vi "CRYProtect All.vi"(8 "sNames":string[](array[string]), 9 "sOption":string, 10 "Index":i32[](array[numeric]), 11 "Type":enum16{"Curves", "Values", "Results", "WFM"}(ring)) -> (0 "Inserted Index":i32[](array[numeric]), 1 "Protect?":bool=TRUE, 2 "Protected Rows":i32[](array[numeric]), 3 "Protected NewNames":string[](array[string]), 4 "Protected OrgNames":string[](array[string]))   [LabVIEW 2013]
uses:
  Global/CRYCurve Library Global.vi
panel:
  # "Prodect All Data(Curves, Values, Results, Waveforms)"
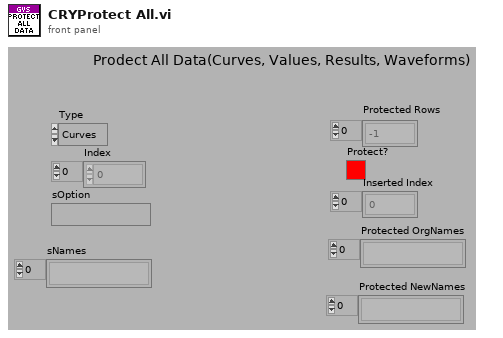
[diagram p1: front panel]
types:
  T1 = enum16{"OK", "Yes", "YesNo", "YesNoCancel", "ReplaceAppend"}
  T2 = cluster{"Curve OrgNames":string[], "Value OrgNames":string[], "Result OrgNames":string[], "WFM OrgNames":string[], "Curve NewNames":string[], "Value NewNames":string[], "Result NewNames":string[], "WFM NewNames":string[]}
  T3 = cluster{"Curve Index":i32[], "Value Index":i32[], "Result Index":i32[], "WFM Index":i32[], "Curve Names":string[], "Value Names":string[], "Result Names":string[], "WFM Names":string[]}
  T4 = typedef "CRYWaveform Cluster Array.ctl" = T5[]
  T5 = typedef "CRYWaveform Cluster.ctl" = cluster{"Waveform":cluster{"X0":dbl, "dX":dbl, "Y":sgl[]}, "X data":u16, "Y data":u16, "Y axis":u16, "X unit":string, "Y unit":string, "Y dB ref":dbl, "display Y":bool, "display X":bool, "Overload?":bool, "Test Info":string, "Step No.":i32, "Name":string, "protected":bool, "Sqc history":string[], "Signal Channel ID":i32, "Plot Settings":cluster{"Color":u32, "Interpolation":u8, "Point Style":u8, "Line Style":u8, "Point Color":u32, "Line Width":u8, "Bar Plot Style":u8, "Fill To":i16}, "AutoProtect":bool}
  T6 = typedef "CRYResult Cluster Array.ctl" = T7[]
  T7 = typedef "CRYResult Cluster.ctl" = cluster{"Name":string, "Margin":dbl, "unit":string, "Verdict":bool, "Limit":string, "Max/Min":string, "protected":bool, "Step No.":i32, "Test Info":string, "AutoProtect":bool}
  T8 = typedef "CRYData Cluster Array.ctl" = T9[]
  T9 = typedef "CRYData Cluster.ctl" = cluster{"Name":string, "Curve":cluster{"x":dbl, "y":dbl, "z":dbl}[], "X data":u16, "Y data":u16, "Z data":u16, "X axis":u16, "Y axis":u16, "Z axis":u16, "X unit":string, "Y unit":string, "Z unit":string, "X dB ref":dbl, "Y dB ref":dbl, "Z dB ref":dbl, "single val":bool, "protected":bool, "display X":bool, "display Y":bool, "display Z":bool, "Test Info":string, "Step No.":i32, "Plot Settings":cluster{"Color":u32, "Interpolation":u8, "Point Style":u8, "Line Style":u8, "Point Color":u32, "Line Width":u8, "Bar Plot Style":u8, "Fill To":i16}, "AutoProtect":bool}
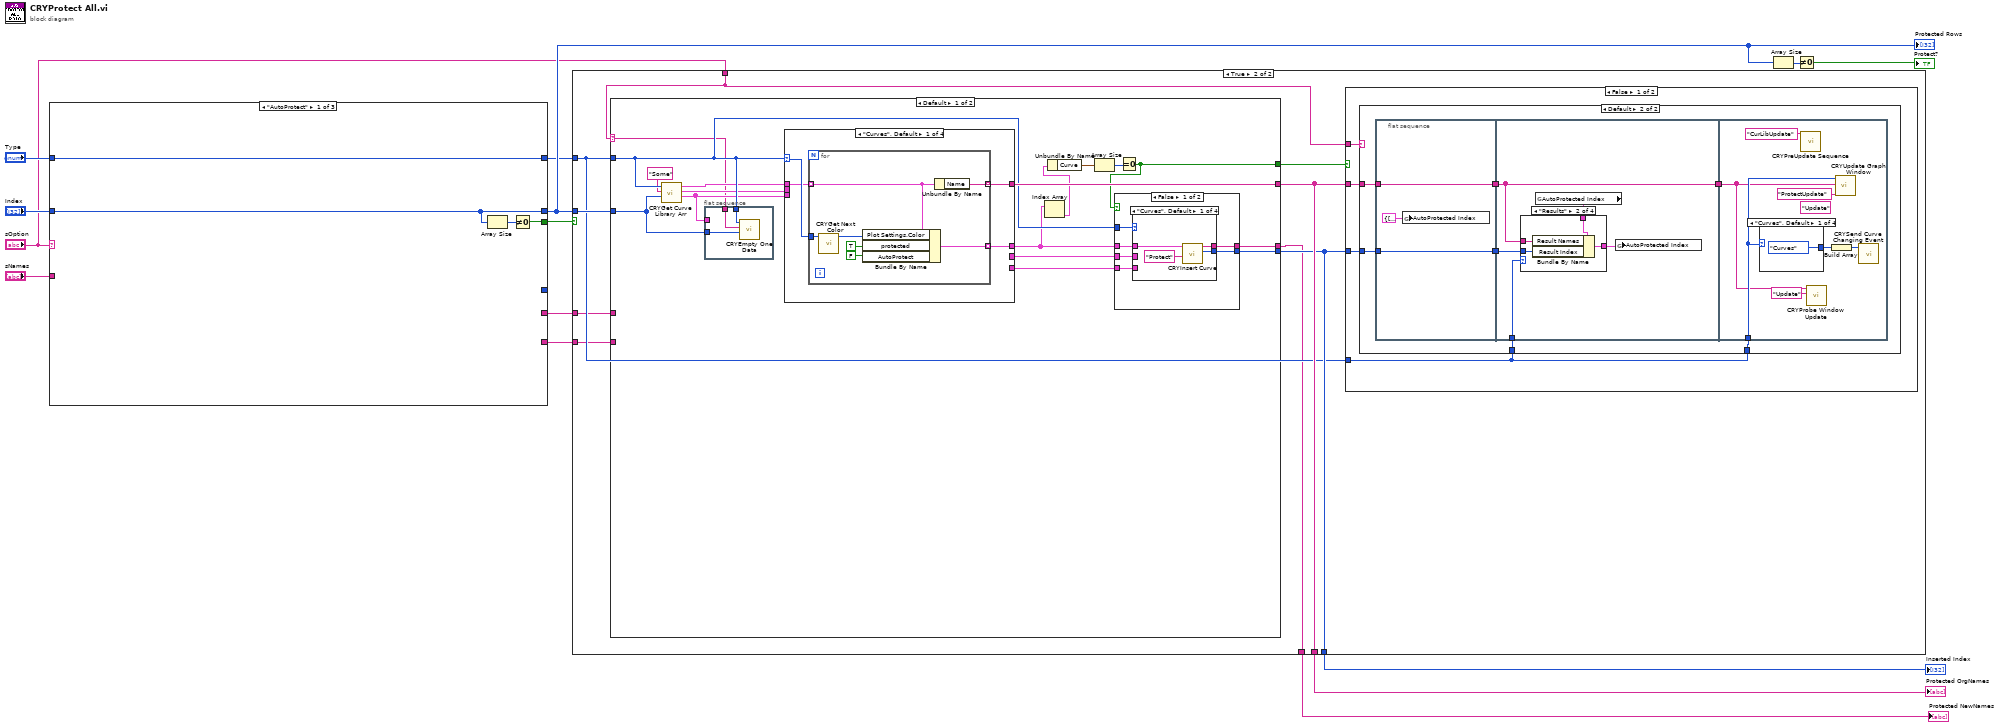
[diagram p0: block diagram]
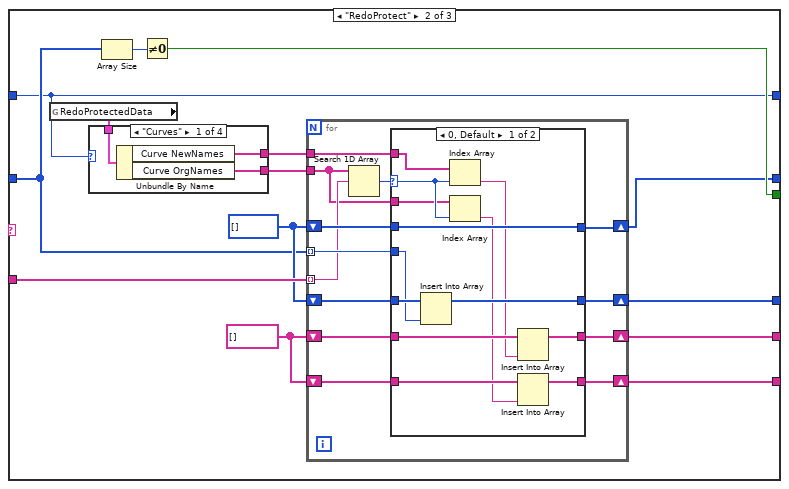
[diagram p2: hidden frame]
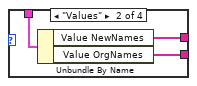
[diagram p3: hidden frame]
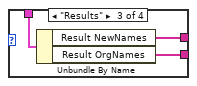
[diagram p4: hidden frame]
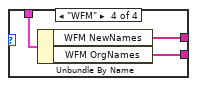
[diagram p5: hidden frame]
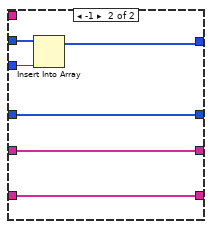
[diagram p6: hidden frame]
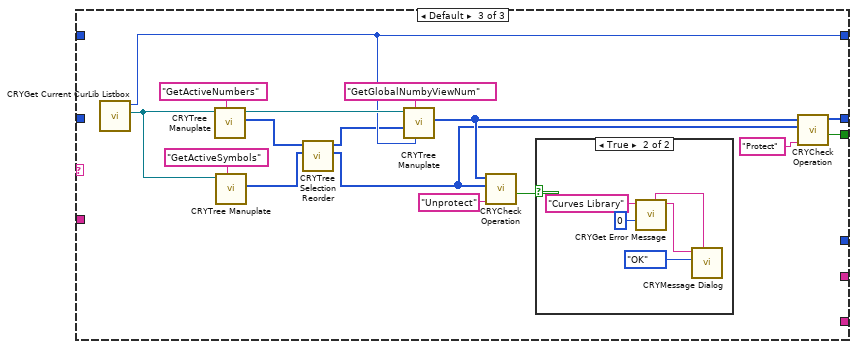
[diagram p7: hidden frame]
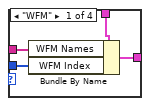
[diagram p11: hidden frame]
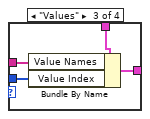
[diagram p12: hidden frame]
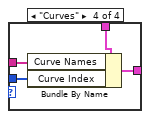
[diagram p13: hidden frame]
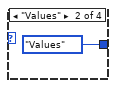
[diagram p14: hidden frame]
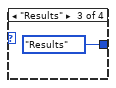
[diagram p15: hidden frame]
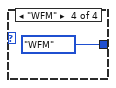
[diagram p16: hidden frame]
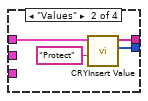
[diagram p18: hidden frame]
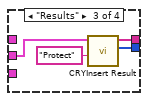
[diagram p19: hidden frame]
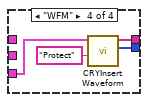
[diagram p20: hidden frame]
diagram:
  n1 = case shown="\"AutoProtect\"" "sOption" {
    tunnel: [w15 w31 w88] -> w14
    tunnel: [w17 w25 w89] -> w13
    tunnel: [w18 w19 w81] -> w10
    tunnel: "Type" -> [w18 w19 _]
    tunnel: "Index" -> [w17 w26 _]
    tunnel: "sNames" -> [_ w28 _]
    tunnel: [_ w24 _] -> _
    tunnel: [_ w23 _] -> w3
    tunnel: [_ w20 _] -> w2
    frame "AutoProtect" {
      n2 = Array Size(array=w17) -> (size(s)=w16:i32)
      n3 = Not Equal To 0?(x=w16) -> (x != 0?=w15:bool)
    }
    frame "RedoProtect" {
      w21 = string[] [] ("sNames")
      w27 = i32[] [] ("Index")
      n4 = global read "CRYCurve Library Global.vi" "RedoProtectedData"() -> (w30:T2)
      n5 = case shown="\"Curves\"" w19 {
        tunnel: w30 -> [w35 w38 w41 w44]
        tunnel: [w34 w37 w40 w43] -> w29
        tunnel: [w33 w36 w39 w42] -> w22
        frame "Curves" {
          n6 = Unbundle By Name(w35) -> ("Curve NewNames"=w33:string[], "Curve OrgNames"=w34:string[])
        }
        frame "Values" {
          n7 = Unbundle By Name(w38) -> ("Value NewNames"=w36:string[], "Value OrgNames"=w37:string[])
        }
        frame "Results" {
          n8 = Unbundle By Name(w41) -> ("Result NewNames"=w39:string[], "Result OrgNames"=w40:string[])
        }
        frame "WFM" {
          n9 = Unbundle By Name(w44) -> ("WFM NewNames"=w42:string[], "WFM OrgNames"=w43:string[])
        }
      }
      n10 = Array Size(array=w26) -> (size(s)=w32:i32)
      n11 = Not Equal To 0?(x=w32) -> (x != 0?=w31:bool)
      n12 = for {
        tunnel: w29 -> [w46]
        tunnel: w28 -> [w49] mode=indexing
        tunnel: w26 -> [w56] mode=indexing
        shift-right: [w54] -> w25
        shift-left: w27 -> [w55]
        shift-right: [w52] -> w24
        shift-left: w27 -> [w53]
        shift-right: [w50] -> w23
        shift-left: w21 -> [w51]
        tunnel: w22 -> [w48]
        shift-right: [w45] -> w20
        shift-left: w21 -> [w47]
        n13 = Search 1D Array(1D array=w46, element=w49) -> (index of element=w57:i32)  [unwired: 1 in]
        n14 = case shown="0, Default" w57 {
          selector: w57 -> [w61 _]
          tunnel: w56 -> [w67 w75]
          tunnel: w55 -> [w70 w76]
          tunnel: [w70 w74] -> w54
          tunnel: w53 -> [w69 w73]
          tunnel: [w68 w73] -> w52
          tunnel: w51 -> [w66 w72]
          tunnel: [w65 w72] -> w50
          tunnel: w48 -> [w64 _]
          tunnel: w47 -> [w62 w71]
          tunnel: w46 -> [w60 _]
          tunnel: [w58 w71] -> w45
          frame 0, Default {
            n15 = Insert Into Array(array=w69, new element=w67) -> (w68:i32[])  [unwired: 1 in]
            n16 = Index Array(array=w64, index=w61) -> (element=w63:string)
            n17 = Index Array(array=w60, index=w61) -> (element=w59:string)
            n18 = Insert Into Array(array=w66, new element=w63) -> (w65:string[])  [unwired: 1 in]
            n19 = Insert Into Array(array=w62, new element=w59) -> (w58:string[])  [unwired: 1 in]
          }
          frame -1 {
            n20 = Insert Into Array(array=w76, new element=w75) -> (w74:i32[])  [unwired: 1 in]
          }
        }
      }
    }
    frame Default {
      n21 = call "CRYGet Current CurLib Listbox.vi"() -> ("CurLib Tree"=w85:refnum<vi>, "Type"=w81:enum16{"Curves", "Values", "Results", "WFM"})  [unwired: 9 in, 1 out]
      n22 = call "CRYTree Manuplate.vi"("sAction"="GetActiveNumbers", "Tree in"=w85) -> ("nData Out"=w80:i32[], "Tree Out"=w83:refnum<vi>)  [unwired: 6 in, 2 out]
      n23 = call "CRYTree Manuplate.vi"("sAction"="GetActiveSymbols", "Tree in"=w85) -> ("nData Out"=w78:i32[])  [unwired: 6 in, 3 out]
      n24 = call "CRYTree Selection Reorder.vi"("Symbol In"=w78, "Number In"=w80) -> ("Symbol Out"=w77:i32[], "Number Out"=w79:i32[])  [unwired: 8 in]
      n25 = call "CRYTree Manuplate.vi"("Type"=w81, "sAction"="GetGlobalNumbyViewNum", "nData"=w79, "Tree in"=w83) -> ("nData Out"=w82:i32[])  [unwired: 4 in, 3 out]
      n26 = call "CRYCheck Operation.vi"("Operation"="Unprotect", "Item Symbols In"=w77, "Index Array In"=w82) -> ("Operation ?"=w92:bool)  [unwired: 6 in, 2 out]
      n27 = case shown="True" w92 {
        frame False {
        }
        frame True {
          n28 = call "CRYGet Error Message.vi"("Error No"=0, "Kind"="Curves Library") -> ("Message"=w94:string, "Window Title"=w93:string)  [unwired: 4 in, 4 out]
          n29 = call "CRYMessage Dialog.vi"("Window Title"=w93, "YesNoCancel"=T1."OK", "Message Content"=w94) -> ()  [unwired: 7 in, 2 out]
        }
      }
      n30 = call "CRYCheck Operation.vi"("Operation"="Protect", "Item Symbols In"=w77, "Index Array In"=w82) -> ("Operation ?"=w88:bool, "Array Out"=w89:i32[])  [unwired: 6 in, 1 out]
    }
  }
  "Protected Rows" <- w13
  n31 = case shown="True" w14 {
    tunnel: w13 -> [_ w106]
    tunnel: w10 -> [_ w103]
    tunnel: "sOption" -> [_ w102]
    tunnel: [_ w104] -> w7
    tunnel: [_ w105] -> w6
    tunnel: w3 -> [_ w101]
    tunnel: w2 -> [_ w100]
    tunnel: [_ w99] -> w1
    frame False {
    }
    frame True {
      n32 = case shown="Default" w102 {
        selector: w102 -> [w159 w245]
        tunnel: w106 -> [w169 w253]
        tunnel: [w168 w234] -> w105
        tunnel: [w167 w235] -> w104
        tunnel: w103 -> [w166 w238]
        tunnel: w101 -> [_ w236]
        tunnel: w100 -> [_ w240]
        tunnel: [w158 w233] -> w99
        tunnel: [w153 _] -> w98
        frame Default {
          n33 = call "CRYGet Curve Library Arr.vi"("Index"=w169, "sOption"="Some", "Type In"=w166) -> ("Waveforms"=w160:T4, "Results"=w164:T6, "Curves/Values"=w165:T8)  [unwired: 6 in]
          n34 = flat-sequence {
            tunnel: w169 -> [w194]
            tunnel: w159 -> [w193]
            tunnel: w166 -> [w192]
            tunnel: w160 -> [_]
            frame #0 {
              n35 = call "CRYEmpty One Data.vi"("Index"=w194, "sOption"=w193, "Type"=w192) -> ()  [unwired: 9 out]
            }
          }
          n36 = case shown="\"Curves\", Default" w166 {
            selector: w166 -> [w197 _ _ w224]
            tunnel: [w198 w208 w216 w225] -> w168
            tunnel: w165 -> [w196 w207 _ _]
            tunnel: w164 -> [_ _ w215 _]
            tunnel: w160 -> [_ _ _ w223]
            tunnel: [w195 w206 _ _] -> w157
            tunnel: [_ _ w214 _] -> w162
            tunnel: [_ _ _ w222] -> w161
            frame "Curves", Default {
              n37 = for {
                tunnel: [w204] -> w198 mode=indexing
                tunnel: w197 -> [w202]
                tunnel: w196 -> [w200] mode=indexing
                tunnel: [w199] -> w195 mode=indexing
                n38 = call "CRYGet Next Color.vi"("Type"=w202) -> ("Color"=w201:u32)  [unwired: 10 out]
                n39 = Bundle By Name(cluster=w200, "Plot Settings.Color"=w201, "protected"=TRUE, "AutoProtect"=FALSE ("protected")) -> (w199:T9)
                n40 = Unbundle By Name(w200) -> ("Name"=w204:string)
              }
            }
            frame "Values" {
              n41 = for {
                tunnel: [w212] -> w208 mode=indexing
                tunnel: w207 -> [w210] mode=indexing
                tunnel: [w209] -> w206 mode=indexing
                n42 = Bundle By Name(cluster=w210, "protected"=TRUE, "AutoProtect"=FALSE) -> (w209:T9)
                n43 = Unbundle By Name(w210) -> ("Name"=w212:string)
              }
            }
            frame "Results" {
              n44 = for {
                tunnel: [w220] -> w216 mode=indexing
                tunnel: w215 -> [w218] mode=indexing
                tunnel: [w217] -> w214 mode=indexing
                n45 = Bundle By Name(cluster=w218, "protected"=TRUE, "AutoProtect"=FALSE) -> (w217:T7)
                n46 = Unbundle By Name(w218) -> ("Name"=w220:string)
              }
            }
            frame "WFM" {
              n47 = for {
                tunnel: [w231] -> w225 mode=indexing
                tunnel: w224 -> [w229]
                tunnel: w223 -> [w227] mode=indexing
                tunnel: [w226] -> w222 mode=indexing
                n48 = call "CRYGet Next Color.vi"("Type"=w229) -> ("Color"=w228:u32)  [unwired: 10 out]
                n49 = Bundle By Name(cluster=w227, "Plot Settings.Color"=w228, "protected"=TRUE, "AutoProtect"=FALSE) -> (w226:T5)
                n50 = Unbundle By Name(w227) -> ("Name"=w231:string)
              }
            }
          }
          n51 = Index Array(array=w157) -> (element=w156:T9)  [unwired: 1 in]
          n52 = Unbundle By Name(w156) -> ("Curve"=w155:cluster{"x":dbl, "y":dbl, "z":dbl}[])
          n53 = Array Size(array=w155) -> (size(s)=w154:i32)
          n54 = Equal To 0?(x=w154) -> (x = 0?=w153:bool)
          n55 = case shown="False" w153 {
            tunnel: [w175 _] -> w167
            tunnel: w166 -> [w174 _]
            tunnel: w162 -> [w173 _]
            tunnel: w161 -> [w172 _]
            tunnel: [w171 _] -> w158
            tunnel: w157 -> [w170 _]
            frame False {
              n56 = case shown="\"Curves\", Default" w174 {
                tunnel: w170 -> [w178 w182 _ _]
                tunnel: [w177 w181 w186 w190] -> w175
                tunnel: w173 -> [_ _ w185 _]
                tunnel: w172 -> [_ _ _ w189]
                tunnel: [w176 w180 w184 w188] -> w171
                frame "Curves", Default {
                  n57 = call "CRYInsert Curve.vi"("sOption"="Protect", "Curve"=w178) -> ("Inserted Index"=w177:i32[], "Inserted Name Out"=w176:string[])  [unwired: 2 in, 6 out]
                }
                frame "Values" {
                  n58 = call "CRYInsert Value.vi"("sOption"="Protect", "Value"=w182) -> ("Inserted Index"=w181:i32[], "Inserted Name Out"=w180:string[])  [unwired: 8 in]
                }
                frame "Results" {
                  n59 = call "CRYInsert Result.vi"("sOption"="Protect", "Result"=w185) -> ("Inserted Index"=w186:i32[], "Inserted Name Out"=w184:string[])  [unwired: 8 in]
                }
                frame "WFM" {
                  n60 = call "CRYInsert Waveform.vi"("sOption"="Protect", "Waveform"=w189) -> ("Inserted Index"=w190:i32[], "Inserted Name Out"=w188:string[])  [unwired: 8 in]
                }
              }
            }
            frame True {
            }
          }
        }
        frame "RedoProtect" {
          n61 = flat-sequence {
            tunnel: w245 -> [w327]
            tunnel: w238 -> [w324]
            tunnel: w240 -> [w326]
            tunnel: w239 -> [_]
            frame #0 {
              n62 = for {
                tunnel: w324 -> [w330]
                tunnel: w326 -> [w329] mode=indexing
                tunnel: [w328] -> w325 mode=indexing
                n63 = call "CRYGet Curve Library One Data .vi"("Data Name"=w329, "Type"=w330) -> ("index"=w328:i32)  [unwired: 3 in, 6 out]
              }
              n64 = call "CRYEmpty One Data.vi"("Index"=w325, "sOption"=w327, "Type"=w324) -> ()  [unwired: 9 out]
            }
          }
          n65 = flat-sequence {
            tunnel: w253 -> [w266]
            tunnel: [w265] -> w234
            tunnel: [w264] -> w235
            tunnel: w245 -> [w256]
            tunnel: w237 -> [w255]
            tunnel: [w254] -> w233
            frame #0 {
              n66 = call "CRYGet Curve Library Arr.vi"("Index"=w266, "sOption"="Some", "Type In"=w255) -> ("Waveforms"=w257:T4, "Results"=w262:T6, "Curves/Values"=w263:T8)  [unwired: 6 in]
              n67 = flat-sequence {
                tunnel: w266 -> [w269]
                tunnel: w256 -> [w268]
                tunnel: w255 -> [w267]
                tunnel: w257 -> [_]
                frame #0 {
                  n68 = call "CRYEmpty One Data.vi"("Index"=w269, "sOption"=w268, "Type"=w267) -> ()  [unwired: 9 out]
                }
              }
              n69 = case shown="\"WFM\"" w255 {
                selector: w255 -> [w272 _ _ w299]
                tunnel: [w273 w283 w291 w300] -> w265
                tunnel: w263 -> [w271 w282 _ _]
                tunnel: w262 -> [_ _ w290 _]
                tunnel: w257 -> [_ _ _ w298]
                tunnel: [w270 w281 _ _] -> w260
                tunnel: [_ _ w289 _] -> w259
                tunnel: [_ _ _ w297] -> w258
                frame "Curves", Default {
                  n70 = for {
                    tunnel: [w279] -> w273 mode=indexing
                    tunnel: w272 -> [w277]
                    tunnel: w271 -> [w275] mode=indexing
                    tunnel: [w274] -> w270 mode=indexing
                    n71 = call "CRYGet Next Color.vi"("Type"=w277) -> ("Color"=w276:u32)  [unwired: 10 out]
                    n72 = Bundle By Name(cluster=w275, "Plot Settings.Color"=w276, "protected"=TRUE, "AutoProtect"=FALSE ("protected")) -> (w274:T9)
                    n73 = Unbundle By Name(w275) -> ("Name"=w279:string)
                  }
                }
                frame "Values" {
                  n74 = for {
                    tunnel: [w287] -> w283 mode=indexing
                    tunnel: w282 -> [w285] mode=indexing
                    tunnel: [w284] -> w281 mode=indexing
                    n75 = Bundle By Name(cluster=w285, "protected"=TRUE, "AutoProtect"=FALSE) -> (w284:T9)
                    n76 = Unbundle By Name(w285) -> ("Name"=w287:string)
                  }
                }
                frame "Results" {
                  n77 = for {
                    tunnel: [w295] -> w291 mode=indexing
                    tunnel: w290 -> [w293] mode=indexing
                    tunnel: [w292] -> w289 mode=indexing
                    n78 = Bundle By Name(cluster=w293, "protected"=TRUE, "AutoProtect"=FALSE) -> (w292:T7)
                    n79 = Unbundle By Name(w293) -> ("Name"=w295:string)
                  }
                }
                frame "WFM" {
                  n80 = for {
                    tunnel: [w306] -> w300 mode=indexing
                    tunnel: w299 -> [w304]
                    tunnel: w298 -> [w302] mode=indexing
                    tunnel: [w301] -> w297 mode=indexing
                    n81 = call "CRYGet Next Color.vi"("Type"=w304) -> ("Color"=w303:u32)  [unwired: 10 out]
                    n82 = Bundle By Name(cluster=w302, "Plot Settings.Color"=w303, "protected"=TRUE, "AutoProtect"=FALSE) -> (w301:T5)
                    n83 = Unbundle By Name(w302) -> ("Name"=w306:string)
                  }
                }
              }
              n84 = case shown="\"WFM\"" w255 {
                tunnel: w260 -> [w310 w314 _ _]
                tunnel: [w309 w313 w318 w322] -> w264
                tunnel: w259 -> [_ _ w317 _]
                tunnel: w258 -> [_ _ _ w321]
                tunnel: [w308 w312 w316 w320] -> w254
                frame "Curves", Default {
                  n85 = call "CRYInsert Curve.vi"("sOption"="Protect", "Curve"=w310) -> ("Inserted Index"=w309:i32[], "Inserted Name Out"=w308:string[])  [unwired: 2 in, 6 out]
                }
                frame "Values" {
                  n86 = call "CRYInsert Value.vi"("sOption"="Protect", "Value"=w314) -> ("Inserted Index"=w313:i32[], "Inserted Name Out"=w312:string[])  [unwired: 8 in]
                }
                frame "Results" {
                  n87 = call "CRYInsert Result.vi"("sOption"="Protect", "Result"=w317) -> ("Inserted Index"=w318:i32[], "Inserted Name Out"=w316:string[])  [unwired: 8 in]
                }
                frame "WFM" {
                  n88 = call "CRYInsert Waveform.vi"("sOption"="Protect", "Waveform"=w321) -> ("Inserted Index"=w322:i32[], "Inserted Name Out"=w320:string[])  [unwired: 8 in]
                }
              }
            }
          }
          n89 = call "CRYGlobal Manipulate.vi"("Type"=w238, "sOption"="byNames", "sAction"="GetGlobal", "sData"=w236) -> ("Curves Out"=w250:T9[], "Values Out"=w249:T9[], "WFM Out"=w247:T5[], "Results Out"=w248:T7[])  [unwired: 5 in, 3 out]
          n90 = call "CRYGlobal Manipulate.vi"("Type"=w238, "sOption"="byNames", "sAction"="GetGlobal", "sData"=w240) -> ("Curves Out"=w243:T9[], "Values Out"=w242:T9[], "WFM Out"=w239:T5[], "Results Out"=w241:T7[])  [unwired: 5 in, 3 out]
          n91 = case shown="\"Curves\", Default" w238 {
            selector: w238 -> [w331 w360 w386 w403]
            tunnel: w250 -> [w337 _ _ _]
            tunnel: w249 -> [_ w358 _ _]
            tunnel: w248 -> [_ _ w385 _]
            tunnel: w247 -> [_ _ _ w402]
            tunnel: w243 -> [w336 _ _ _]
            tunnel: w242 -> [_ w357 _ _]
            tunnel: w241 -> [_ _ w384 _]
            tunnel: w239 -> [_ _ _ w401]
            tunnel: w236 -> [w333 w361 w387 w404]
            tunnel: [w331 w360 w386 w403] -> w237
            frame "Curves", Default {
              n92 = for {
                tunnel: w337 -> [w340] mode=indexing
                tunnel: [w339] -> w332 mode=indexing
                tunnel: w336 -> [w338] mode=indexing
                n93 = Unbundle By Name(w338) -> ("Curve"=w356:cluster{"x":dbl, "y":dbl, "z":dbl}[], "X data"=w355:u16, "Y data"=w354:u16, "Z data"=w353:u16, "X axis"=w352:u16, "Y axis"=w351:u16, "Z axis"=w350:u16, "X unit"=w349:string, "Y unit"=w348:string, "Z unit"=w347:string, "X dB ref"=w346:dbl, "Y dB ref"=w345:dbl, "Z dB ref"=w344:dbl, "display X"=w343:bool, "display Y"=w342:bool, "display Z"=w341:bool)
                n94 = Bundle By Name(cluster=w340, "Curve"=w356, "X data"=w355, "Y data"=w354, "Z data"=w353, "X axis"=w352, "Y axis"=w351, "Z axis"=w350, "X unit"=w349, "Y unit"=w348, "Z unit"=w347, "X dB ref"=w346, "Y dB ref"=w345, "Z dB ref"=w344, "display X"=w343, "display Y"=w342, "display Z"=w341) -> (w339:T9)
              }
              n95 = call "CRYGlobal Manipulate.vi"("Type"=w331, "sOption"="byNames", "sAction"="Replace", "sData"=w333, "Curves"=w332) -> ()  [unwired: 4 in, 7 out]
            }
            frame "Values" {
              n96 = for {
                tunnel: w358 -> [w366] mode=indexing
                tunnel: [w365] -> w359 mode=indexing
                tunnel: w357 -> [w364] mode=indexing
                n97 = Unbundle By Name(w364) -> ("Curve"=w382:cluster{"x":dbl, "y":dbl, "z":dbl}[], "X data"=w381:u16, "Y data"=w380:u16, "Z data"=w379:u16, "X axis"=w378:u16, "Y axis"=w377:u16, "Z axis"=w376:u16, "X unit"=w375:string, "Y unit"=w374:string, "Z unit"=w373:string, "X dB ref"=w372:dbl, "Y dB ref"=w371:dbl, "Z dB ref"=w370:dbl, "display X"=w369:bool, "display Y"=w368:bool, "display Z"=w367:bool)
                n98 = Bundle By Name(cluster=w366, "Curve"=w382, "X data"=w381, "Y data"=w380, "Z data"=w379, "X axis"=w378, "Y axis"=w377, "Z axis"=w376, "X unit"=w375, "Y unit"=w374, "Z unit"=w373, "X dB ref"=w372, "Y dB ref"=w371, "Z dB ref"=w370, "display X"=w369, "display Y"=w368, "display Z"=w367) -> (w365:T9)
              }
              n99 = call "CRYGlobal Manipulate.vi"("Type"=w360, "sOption"="byNames", "sAction"="Replace", "sData"=w361, "Values"=w359) -> ()  [unwired: 4 in, 7 out]
            }
            frame "Results" {
              n100 = for {
                tunnel: w385 -> [w399] mode=indexing
                tunnel: [w398] -> w383 mode=indexing
                tunnel: w384 -> [w397] mode=indexing
                n101 = Unbundle By Name(w397) -> ("Margin"=w396:dbl, "unit"=w395:string, "Verdict"=w394:bool, "Limit"=w393:string, "Max/Min"=w392:string, "Step No."=w391:i32, "Test Info"=w390:string)
                n102 = Bundle By Name(cluster=w399, "Margin"=w396, "unit"=w395, "Verdict"=w394, "Limit"=w393, "Max/Min"=w392, "Step No."=w391, "Test Info"=w390) -> (w398:T7)
              }
              n103 = call "CRYGlobal Manipulate.vi"("Type"=w386, "sOption"="byNames", "sAction"="Replace", "sData"=w387, "Results"=w383) -> ()  [unwired: 4 in, 7 out]
            }
            frame "WFM" {
              n104 = for {
                tunnel: w402 -> [w423] mode=indexing
                tunnel: [w422] -> w400 mode=indexing
                tunnel: w401 -> [w421] mode=indexing
                n105 = Unbundle By Name(w421) -> ("Waveform"=w420:cluster{"X0":dbl, "dX":dbl, "Y":sgl[]}, "X data"=w419:u16, "Y data"=w418:u16, "Y axis"=w417:u16, "X unit"=w416:string, "Y unit"=w415:string, "Y dB ref"=w414:dbl, "display Y"=w413:bool, "display X"=w412:bool, "Overload?"=w411:bool, "Test Info"=w410:string, "Step No."=w409:i32, "Sqc history"=w408:string[], "Signal Channel ID"=w407:i32)
                n106 = Bundle By Name(cluster=w423, "Waveform"=w420, "X data"=w419, "Y data"=w418, "Y axis"=w417, "X unit"=w416, "Y unit"=w415, "Y dB ref"=w414, "display Y"=w413, "display X"=w412, "Overload?"=w411, "Test Info"=w410, "Step No."=w409, "Sqc history"=w408, "Signal Channel ID"=w407) -> (w422:T5)
              }
              n107 = call "CRYGlobal Manipulate.vi"("Type"=w403, "sOption"="byNames", "sAction"="Replace", "sData"=w404, "WFM"=w400) -> ()  [unwired: 4 in, 7 out]
            }
          }
        }
      }
      n108 = case shown="False" w98 {
        tunnel: w105 -> [w110 _]
        tunnel: w104 -> [w109 _]
        tunnel: w103 -> [w108 _]
        tunnel: w102 -> [w107 _]
        frame False {
          n109 = case shown="Default" w107 {
            tunnel: w110 -> [_ w117]
            tunnel: w109 -> [_ w115]
            tunnel: w108 -> [_ w112]
            tunnel: w108 -> [_ w111]
            frame "AutoProtect", "RedoProtect" {
              # "In Sequence Run or Redo , donot update curvelibgraph"
            }
            frame Default {
              n110 = flat-sequence {
                tunnel: w115 -> [w119]
                tunnel: w117 -> [w120]
                tunnel: [w120] -> w114
                tunnel: [w119] -> w113
                tunnel: [w121] -> w116
                tunnel: w114 -> [w121]
                tunnel: w113 -> [w123]
                tunnel: w111 -> [w122]
                tunnel: w116 -> [w142]
                tunnel: w112 -> [w143]
                frame #0 {
                  n111 = global write "CRYCurve Library Global.vi" "AutoProtected Index"(T3 {"Curve Index"=[], "Value Index"=[], "Result Index"=[], "WFM Index"=[], "Curve Names"=[], "Value Names"=[], "Result Names"=[], "WFM Names"=[]} ("AutoProtected Index")) -> ()
                }
                frame #1 {
                  n112 = global read "CRYCurve Library Global.vi" "AutoProtected Index"() -> (w125:T3)
                  n113 = case shown="\"Results\"" w122 {
                    tunnel: w125 -> [w129 w133 w137 w141]
                    tunnel: [w128 w132 w136 w140] -> w124
                    tunnel: w123 -> [w126 w130 w134 w138]
                    tunnel: w121 -> [w127 w131 w135 w139]
                    frame "WFM" {
                      n114 = Bundle By Name(cluster=w129, "WFM Names"=w127, "WFM Index"=w126) -> (w128:T3)
                    }
                    frame "Results" {
                      n115 = Bundle By Name(cluster=w133, "Result Names"=w131, "Result Index"=w130) -> (w132:T3)
                    }
                    frame "Values" {
                      n116 = Bundle By Name(cluster=w137, "Value Names"=w135, "Value Index"=w134) -> (w136:T3)
                    }
                    frame "Curves" {
                      n117 = Bundle By Name(cluster=w141, "Curve Names"=w139, "Curve Index"=w138) -> (w140:T3)
                    }
                  }
                  n118 = global write "CRYCurve Library Global.vi" "AutoProtected Index"(w124) -> ()
                }
                frame #2 {
                  (unwired) "Update" ("sOption")
                  n119 = case shown="\"Curves\", Default" w143 {
                    tunnel: [enum16{"Curves", "Values", "Results", "WFM"}."Curves" ("Type In") enum16{"Curves", "Values", "Results", "WFM"}."Values" ("Type In") enum16{"Curves", "Values", "Results", "WFM"}."Results" ("Type In") enum16{"Curves", "Values", "Results", "WFM"}."WFM" ("Type In")] -> w146
                    frame "Curves", Default {
                    }
                    frame "Values" {
                    }
                    frame "Results" {
                    }
                    frame "WFM" {
                    }
                  }
                  n120 = call "CRYPreUpdate Sequence.vi"("EventName"="CurLibUpdate") -> ()  [unwired: 15 in]
                  n121 = call "CRYProbe Window Update.vi"("sAction"="Update", "Names"=w142) -> ()  [unwired: 2 in, 8 out]
                  n122 = Build Array(w146) -> (w145:enum16{"Curves", "Values", "Results", "WFM"}[])
                  n123 = call "CRYUpdate Graph Window.vi"("sOption"="ProtectUpdate", "Del/Update Names"=w142, "Type"=w143) -> ()  [unwired: 1 in, 8 out]
                  n124 = call "CRYSend Curve Changing Event.vi"("Type"=w145) -> ()  [unwired: 11 out]
                }
              }
            }
          }
        }
        frame True {
        }
      }
    }
  }
  "Inserted Index" <- w7
  "Protected OrgNames" <- w6
  "Protected NewNames" <- w1
  n125 = Array Size(array=w13) -> (size(s)=w12:i32)
  n126 = Not Equal To 0?(x=w12) -> (x != 0?=→"Protect?":bool)
